vi "TestDataBase.vi"() -> ()   [LabVIEW 2024]
uses:
  Controls/DataBaseControl.ctl
  <vilib>/addons/database/Auxilliary.llb/DB Tools Column Info.ctl
  <vilib>/addons/database/Auxilliary.llb/DB Tools DataTypes.ctl
  <vilib>/addons/database/Connection.llb/DB Tools Open Connec (String).vi
  <vilib>/addons/database/NI_Database_API.lvlib
  <vilib>/addons/database/_DB Variant To Data/Database Variant To Data.xnode
panel:
  in  "Function":u16(ring) items=["Create Only", "Create and Insert (With Names)", "Create and Insert (Generic Names)", "Delete Table"]
  in  "column information":T1[](array[typedef])=[{"column name"="stringcol", "data type"=enum."String", "size"=50, "allow null?"=FALSE}, {"column name"="intcol", "data type"=enum."Long (I32)", "size"=0, "allow null?"=TRUE}, {"column name"="doublecol", "data type"=enum."Double (DBL)", "size"=0, "allow null?"=TRUE}]
  in  "sample data":T3={"String"="This is a test string", "Numeric"=101, "Numeric 2"=3.14}
  in  "Table":string="createtable"
  out "Database Information":string[][](table)
  out "String 2":string
  out "size(s) 3":i32
  out "size(s) 2":i32
  out "size(s)":i32
  out "data":T1[](array[typedef])
  in  "?":T4
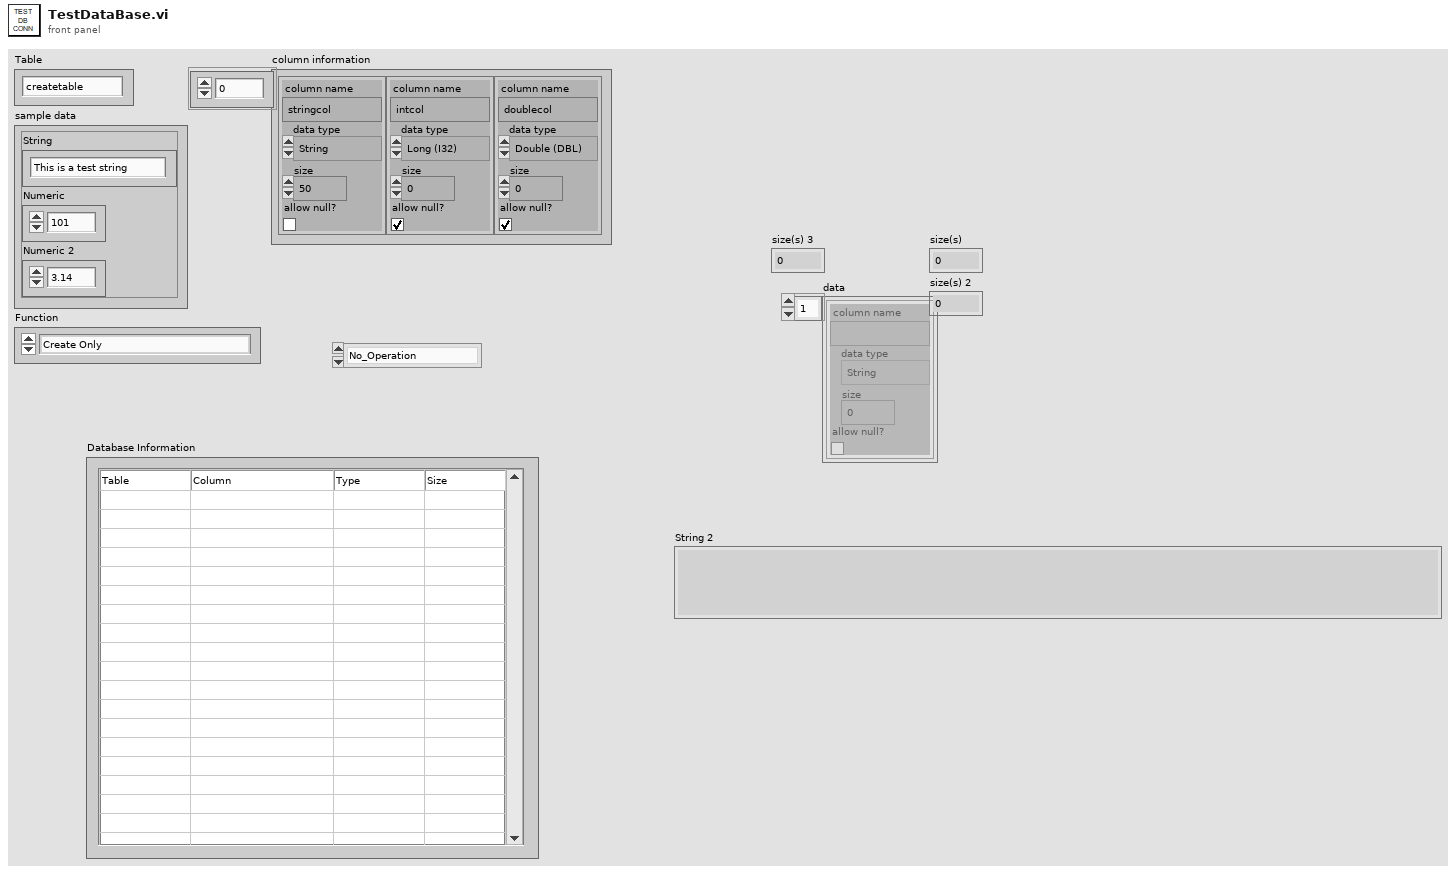
[diagram p1: front panel]
types:
  T1 = typedef "NI_Database_API.lvlib/DB Tools Column Info.ctl" = cluster{"column name":string, "data type":T2, "size":i32, "allow null?":bool}
  T2 = typedef "NI_Database_API.lvlib/DB Tools DataTypes.ctl" = enum16{"String", "Long (I32)", "Single (SGL)", "Double (DBL)", "Date/Time", "Binary"}
  T3 = cluster{"String":string, "Numeric":i32, "Numeric 2":dbl}
  T4 = typedef "DataBaseControl.ctl" = enum16{"No_Operation", "Table_Delete", "Table_Create", "AppendData", "ReadData", "TableColumn"}
  T5 = typedef "NI_Database_API.lvlib/Conn ObjectReference.ctl" = refnum<k1>
  T6 = cluster{"name":string, "database data type":T2, "defined size":i32}[]
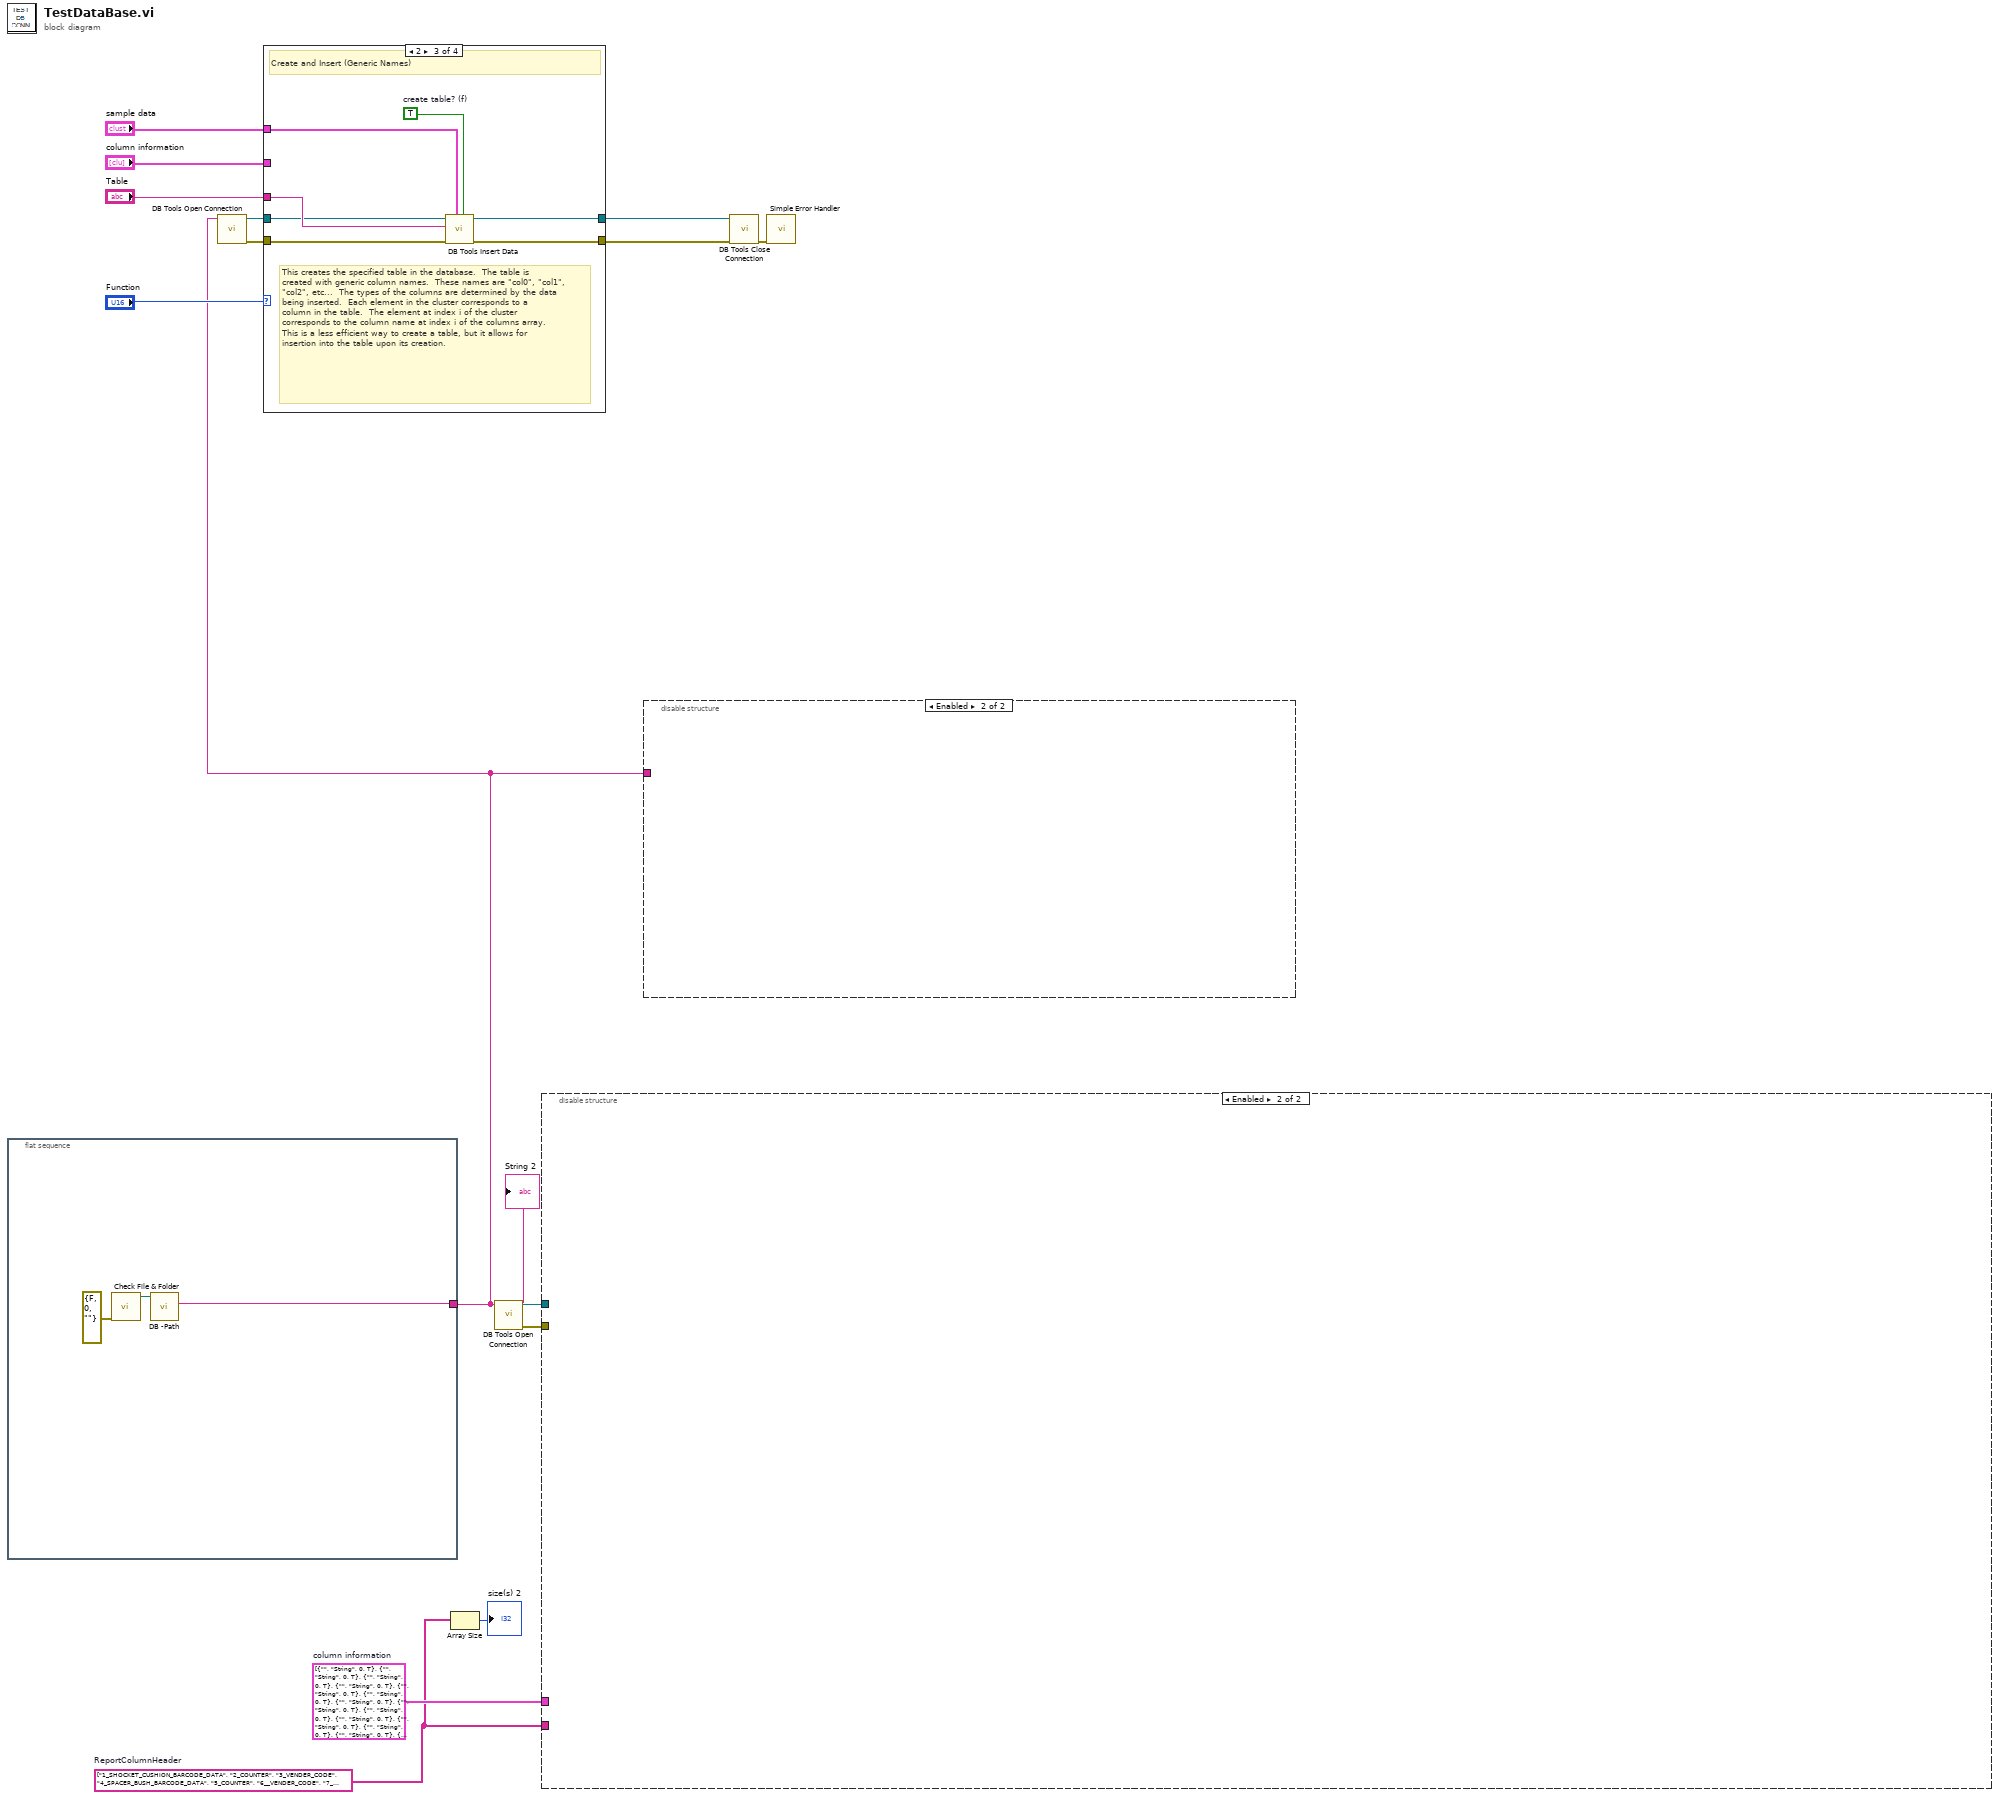
[diagram p0: block diagram]
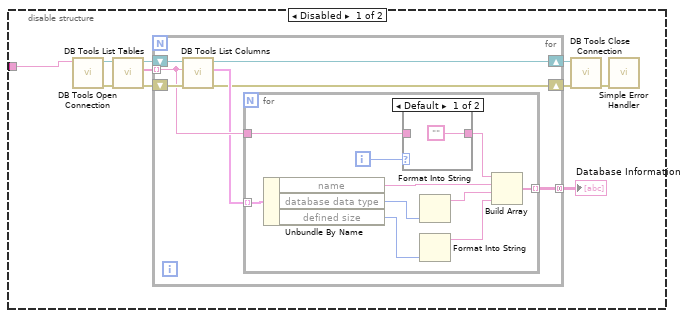
[diagram p2: hidden frame]
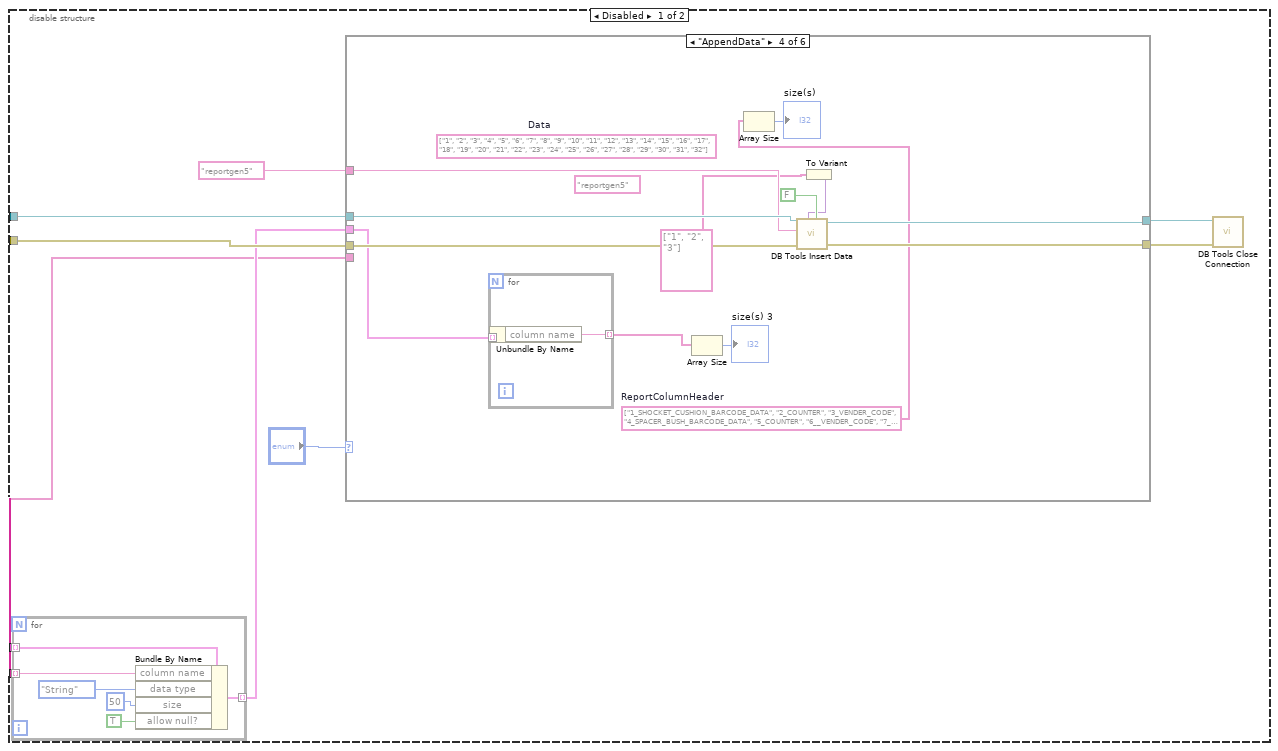
[diagram p4: hidden frame]
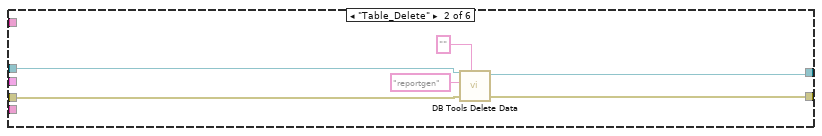
[diagram p6: hidden frame]
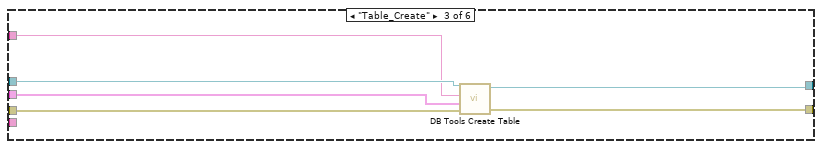
[diagram p7: hidden frame]
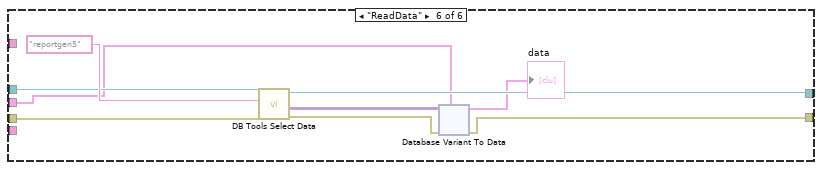
[diagram p9: hidden frame]
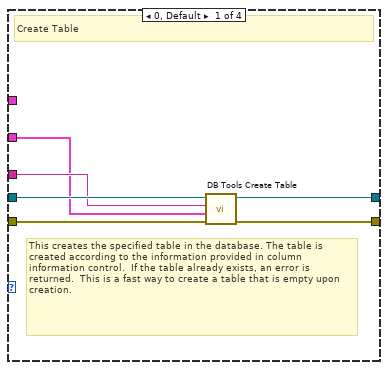
[diagram p10: hidden frame]
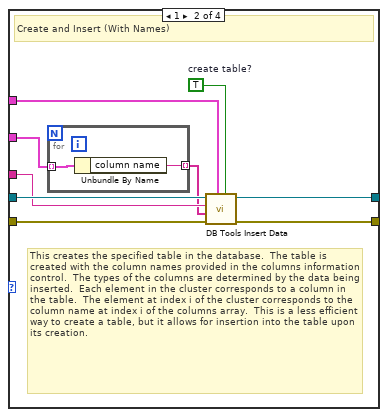
[diagram p11: hidden frame]
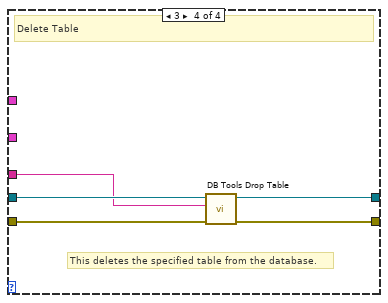
[diagram p12: hidden frame]
diagram:
  w12 = string[] ["1_SHOCKET_CUSHION_BARCODE_DATA", "2_COUNTER", "3_VENDER_CODE", "4_SPACER_BUSH_BARCODE_DATA", "5_COUNTER", "6__VENDER_CODE", "7_COUNTER", "8_VENDER_CODE", "9_SILENT_BLOCK_BARCODE_DATA", "10_COUNTER", "11_VENDER_CODE", "12_ARNLOCK_WARCEL_BARCODE_DATA", "13_COUNTER", "14_VENDER_CODE", "15_BELL_CRANK", "16_COUNTER", "17_VENDER_CODE", "18_FIX_BV3_BX4ATION_SHAFT_BARCODE_DATA", "19_COUNTER", "20_VENDER_CODE", "21_SPRING_BARCODE_DATA", "22_COUNTER", "23_VENDER_CODE", "24_KNOB_BARCODE_DATA", "25_COUNTER", "26_VENDER_CODE", "27_DELUX_BARCODE_DATA", "28_COUNTER", "29_VENDER_CODE", "30_INSERT_LOCK_BARCODE_DATA", "31_COUNTER", "32_VENDER_CODE"]  # ReportColumnHeader
  w13 = T1[] [{"column name"="", "data type"=enum."String", "size"=0, "allow null?"=TRUE}, {"column name"="", "data type"=enum."String", "size"=0, "allow null?"=TRUE}, {"column name"="", "data type"=enum."String", "size"=0, "allow null?"=TRUE}, {"column name"="", "data type"=enum."String", "size"=0, "allow null?"=TRUE}, {"column name"="", "data type"=enum."String", "size"=0, "allow null?"=TRUE}, {"column name"="", "data type"=enum."String", "size"=0, "allow null?"=TRUE}, {"column name"="", "data type"=enum."String", "size"=0, "allow null?"=TRUE}, {"column name"="", "data type"=enum."String", "size"=0, "allow null?"=TRUE}, {"column name"="", "data type"=enum."String", "size"=0, "allow null?"=TRUE}, {"column name"="", "data type"=enum."String", "size"=0, "allow null?"=TRUE}, {"column name"="", "data type"=enum."String", "size"=0, "allow null?"=TRUE}, {"column name"="", "data type"=enum."String", "size"=0, "allow null?"=TRUE}, {"column name"="", "data type"=enum."String", "size"=0, "allow null?"=TRUE}, {"column name"="", "data type"=enum."String", "size"=0, "allow null?"=TRUE}, {"column name"="", "data type"=enum."String", "size"=0, "allow null?"=TRUE}, {"column name"="", "data type"=enum."String", "size"=0, "allow null?"=TRUE}, {"column name"="", "data type"=enum."String", "size"=0, "allow null?"=TRUE}, {"column name"="", "data type"=enum."String", "size"=0, "allow null?"=TRUE}, {"column name"="", "data type"=enum."String", "size"=0, "allow null?"=TRUE}, {"column name"="", "data type"=enum."String", "size"=0, "allow null?"=TRUE}, {"column name"="", "data type"=enum."String", "size"=0, "allow null?"=TRUE}, {"column name"="", "data type"=enum."String", "size"=0, "allow null?"=TRUE}, {"column name"="", "data type"=enum."String", "size"=0, "allow null?"=TRUE}, {"column name"="", "data type"=enum."String", "size"=0, "allow null?"=TRUE}, {"column name"="", "data type"=enum."String", "size"=0, "allow null?"=TRUE}, {"column name"="", "data type"=enum."String", "size"=0, "allow null?"=TRUE}, {"column name"="", "data type"=enum."String", "size"=0, "allow null?"=TRUE}, {"column name"="", "data type"=enum."String", "size"=0, "allow null?"=TRUE}, {"column name"="", "data type"=enum."String", "size"=0, "allow null?"=TRUE}, {"column name"="", "data type"=enum."String", "size"=0, "allow null?"=TRUE}, {"column name"="", "data type"=enum."String", "size"=0, "allow null?"=TRUE}, {"column name"="", "data type"=enum."String", "size"=0, "allow null?"=TRUE}]  # column information
  n1 = flat-sequence {
    tunnel: [w16] -> w1
    frame #0 {
      n2 = call "Check File & Folder .vi"("error in (no error)"=errorcluster {"status"=FALSE, "code"=0, "source"=""}) -> ("Config Path"=w17:path)  [unwired: 8 in, 2 out]
      n3 = call "DB -Path.vi"("path"=w17) -> ("String 2"=w16:string)  [unwired: 8 in, 2 out]
    }
  }
  n4 = call-poly <vilib>:"DB Tools Open Connection.vi"("connection information"=w1) -> ("error out"=w6:errorcluster, "connection reference"=w7:T5)  [unwired: 7 in]
  n5 = case shown="2" "Function" {
    tunnel: w7 -> [w24 w33 w37 w47]
    tunnel: w6 -> [w23 w30 w38 w46]
    tunnel: "Table" -> [w22 w27 w39 w43]
    tunnel: [w21 w28 w40 w45] -> w9
    tunnel: [w20 w29 w42 w44] -> w8
    tunnel: "sample data" -> [_ w31 w36 _]
    tunnel: "column information" -> [w19 w26 _ _]
    frame 0, Default {
      # "This creates the specified table in the database. The table is created according to the information provided in column information control.  If the table already exists, an error is returned.  This is a fast way to create a table that is empty upon creation."
      # "Create Table"
      n6 = call <vilib>:"DB Tools Create Table.vi"("error in (no error)"=w23, "column information"=w19, "table"=w22, "connection reference"=w24) -> ("error out"=w20:errorcluster, "connection reference out"=w21:T5)  [unwired: 4 in]
    }
    frame 1 {
      w32 = TRUE  # create table?
      # "This creates the specified table in the database.  The table is created with the column names provided in the columns information control.  The types of the columns are determined by the data being inserted.  Each element in the cluster corresponds to a column in the table.  The element at index i of the cluster corresponds to the column name at index i of the columns array.  This is a less efficient way to create a table, but it allows for insertion into the table upon its creation."
      # "Create and Insert (With Names)"
      n7 = for {
        tunnel: w26 -> [w35] mode=indexing
        tunnel: [w34] -> w25 mode=indexing
        n8 = Unbundle By Name(w35) -> ("column name"=w34:string)
      }
      n9 = call <vilib>:"DB Tools Insert Data.vi"("create table? (F)"=w32, "data"=w31, "error in (no error)"=w30, "columns"=w25, "table"=w27, "connection reference"=w33) -> ("error out"=w29:errorcluster, "connection reference out"=w28:T5)  [unwired: 4 in]
    }
    frame 2 {
      w41 = TRUE  # create table? (f)
      # "This creates the specified table in the database.  The table is created with generic column names.  These names are \"col0\", \"col1\", \"col2\", etc...  The types of the columns are determined by the data being inserted.  Each element in the cluster corresponds to a column in the table.  The element at index i of the cluster corresponds to the column name at index i of the columns array.  This is a less efficient way to create a table, but it allows for insertion into the table upon its creation."
      # "Create and Insert (Generic Names)"
      n10 = call <vilib>:"DB Tools Insert Data.vi"("create table? (F)"=w41, "data"=w36, "error in (no error)"=w38, "table"=w39, "connection reference"=w37) -> ("error out"=w42:errorcluster, "connection reference out"=w40:T5)  [unwired: 5 in]
    }
    frame 3 {
      # "This deletes the specified table from the database."
      # "Delete Table"
      n11 = call <vilib>:"DB Tools Drop Table.vi"("error in (no error)"=w46, "table"=w43, "connection reference"=w47) -> ("error out"=w44:errorcluster, "connection reference out"=w45:T5)  [unwired: 5 in]
    }
  }
  n12 = Array Size(array=w12) -> (size(s)=→"size(s) 2":i32)
  n13 = call-poly <vilib>:"DB Tools Open Connection.vi"("connection information"=w1) -> ("error out"=w15:errorcluster, "connection reference"=w14:T5)  [unwired: 7 in]
  n14 = disable-structure shown="Enabled" {
    disable-tunnel: w15 -> [w55 _]
    disable-tunnel: w14 -> [w54 _]
    disable-tunnel: w13 -> [w51 _]
    disable-tunnel: w12 -> [w48 _]
    frame Disabled {
      n15 = for {
        tunnel: w51 -> [w236] mode=indexing
        tunnel: w48 -> [w234] mode=indexing
        tunnel: [w231] -> w50 mode=indexing
        n16 = Bundle By Name(cluster=w236, "column name"=w234, "data type"=DB_Tools_DataTypes."String", "size"=50, "allow null?"=TRUE) -> (w231:T1)
      }
      n17 = case shown="\"AppendData\"" "?" {
        tunnel: w55 -> [w57 w62 w70 w78 w87 w95]
        tunnel: w54 -> [w58 w61 w69 w83 w86 w94]
        tunnel: [w57 w60 w68 w82 w87 w89] -> w53
        tunnel: [w58 w59 w67 w81 w86 w93] -> w52
        tunnel: w50 -> [_ _ w66 w77 _ w91]
        tunnel: w48 -> [_ _ _ _ _ _]
        tunnel: "reportgen5" ("table") -> [_ _ w65 w79 _ _]
        frame "No_Operation", Default {
        }
        frame "Table_Delete" {
          n18 = call <vilib>:"DB Tools Delete Data.vi"("condition"="", "error in (no error)"=w62, "table"="reportgen", "connection reference"=w61) -> ("error out"=w60:errorcluster, "connection reference out"=w59:T5)  [unwired: 6 in]
        }
        frame "Table_Create" {
          n19 = call <vilib>:"DB Tools Create Table.vi"("error in (no error)"=w70, "column information"=w66, "table"=w65, "connection reference"=w69) -> ("error out"=w68:errorcluster, "connection reference out"=w67:T5)  [unwired: 4 in]
        }
        frame "AppendData" {
          w76 = string[] ["1_SHOCKET_CUSHION_BARCODE_DATA", "2_COUNTER", "3_VENDER_CODE", "4_SPACER_BUSH_BARCODE_DATA", "5_COUNTER", "6__VENDER_CODE", "7_COUNTER", "8_VENDER_CODE", "9_SILENT_BLOCK_BARCODE_DATA", "10_COUNTER", "11_VENDER_CODE", "12_ARNLOCK_WARCEL_BARCODE_DATA", "13_COUNTER", "14_VENDER_CODE", "15_BELL_CRANK", "16_COUNTER", "17_VENDER_CODE", "18_FIX_BV3_BX4ATION_SHAFT_BARCODE_DATA", "19_COUNTER", "20_VENDER_CODE", "21_SPRING_BARCODE_DATA", "22_COUNTER", "23_VENDER_CODE", "24_KNOB_BARCODE_DATA", "25_COUNTER", "26_VENDER_CODE", "27_DELUX_BARCODE_DATA", "28_COUNTER", "29_VENDER_CODE", "30_INSERT_LOCK_BARCODE_DATA", "31_COUNTER", "32_VENDER_CODE"]  # ReportColumnHeader
          (unwired) string[] ["1", "2", "3", "4", "5", "6", "7", "8", "9", "10", "11", "12", "13", "14", "15", "16", "17", "18", "19", "20", "21", "22", "23", "24", "25", "26", "27", "28", "29", "30", "31", "32"]  # Data
          (unwired) "reportgen5" ("table")
          n20 = for {
            tunnel: w77 -> [w85] mode=indexing
            tunnel: [w84] -> w74 mode=indexing
            n21 = Unbundle By Name(w85) -> ("column name"=w84:string)
          }
          n22 = Array Size(array=w74) -> (size(s)=→"size(s) 3":i32)
          n23 = Array Size(array=w76) -> (size(s)=→"size(s)":i32)
          n24 = To Variant(anything=string[] ["1", "2", "3"] ("columns")) -> (Variant=w72:variant)
          n25 = call <vilib>:"DB Tools Insert Data.vi"("create table? (F)"=FALSE, "data"=w72, "error in (no error)"=w78, "table"=w79, "connection reference"=w83) -> ("error out"=w82:errorcluster, "connection reference out"=w81:T5)  [unwired: 5 in]
        }
        frame "TableColumn" {
        }
        frame "ReadData" {
          n26 = call <vilib>:"DB Tools Select Data.vi"("error in (no error)"=w95, "table"="reportgen5", "connection reference"=w94) -> ("error out"=w90:errorcluster, "data"=w92:variant[][], "connection reference out"=w93:T5)  [unwired: 3 in]
          n27 = xnode "Database Variant To Data"("database variant"=w92, "error in (no error)"=w90, "type"=w91) -> ("data"=→"data":T1[], "error out"=w89:errorcluster)
        }
      }
      n28 = call <vilib>:"DB Tools Close Connection.vi"("error in (no error)"=w53, "connection reference"=w52) -> ()  [unwired: 5 in, 1 out]
    }
    frame Enabled {
    }
  }
  n29 = disable-structure shown="Enabled" {
    disable-tunnel: w1 -> [w237 _]
    frame Disabled {
      n30 = call-poly <vilib>:"DB Tools Open Connection.vi"("connection information"=w237) -> ("error out"=w246:errorcluster, "connection reference"=w245:T5)  [unwired: 7 in]
      n31 = call <vilib>:"DB Tools List Tables.vi"("error in (no error)"=w246, "connection reference"=w245) -> ("error out"=w243:errorcluster, "tables"=w242:string[], "connection reference out"=w244:T5)  [unwired: 3 in]
      n32 = for {
        shift-right: [w249] -> w241
        shift-left: w243 -> [w253]
        tunnel: w242 -> [w251] mode=indexing
        shift-right: [w248] -> w240
        shift-left: w244 -> [w252]
        tunnel: [w247] -> w238 mode=concatenating
        n33 = call <vilib>:"DB Tools List Columns.vi"("error in (no error)"=w253, "table"=w251, "connection reference"=w252) -> ("error out"=w249:errorcluster, "column information"=w250:T6, "connection reference out"=w248:T5)  [unwired: 1 in, 1 out]
        n34 = for {
          tunnel: w251 -> [w262]
          tunnel: w250 -> [w259] mode=indexing
          tunnel: [w261] -> w247 mode=indexing
          i -> [w263]
          n35 = Unbundle By Name(w259) -> ("name"=w258:string, "database data type"=w257:T2, "defined size"=w255:i32)
          n36 = case shown="Default" w263 {
            tunnel: w262 -> [_ w265]
            tunnel: ["" w265] -> w260
            frame Default {
            }
            frame 0 {
            }
          }
          n37 = Format Into String(w257) -> (resulting string=w256:string)  [unwired: 3 in, 1 out]
          n38 = Format Into String(w255) -> (resulting string=w254:string)  [unwired: 3 in, 1 out]
          n39 = Build Array(w260, w258, w256, w254) -> (w261:string[])
        }
      }
      "Database Information" <- w238
      n40 = call <vilib>:"DB Tools Close Connection.vi"("error in (no error)"=w241, "connection reference"=w240) -> ("error out"=w239:errorcluster)  [unwired: 5 in]
      n41 = call <vilib>:"Simple Error Handler.vi"("error in (no error)"=w239) -> ()  [unwired: 4 in, 5 out]
    }
    frame Enabled {
    }
  }
  n42 = call <vilib>:"DB Tools Close Connection.vi"("error in (no error)"=w8, "connection reference"=w9) -> ("error out"=w4:errorcluster)  [unwired: 5 in]
  n43 = call <vilib>:"Simple Error Handler.vi"("error in (no error)"=w4) -> ()  [unwired: 4 in, 5 out]
  "String 2" <- w1
